vi "TDMS File Initialization (Write).vi"(8 "error in (no error)":errorcluster, 9 "Write Settings":T4={"Asynchronous"=FALSE, "Disable Buffering if Supported"=FALSE, "Reserved Images"=1000, "Fail if Reservation Fails"=FALSE}, 10 "Image In":T5, 11 "File Path":path) -> (0 "error out":errorcluster, 1 "Write Settings Out":T3 {"Image Type" items=["Grayscale (U8)", "Grayscale (I16)", "Grayscale (SGL)", "Complex (CSG)", "RGB (U32)", "HSL (U32)", "RGB (U64)", "Grayscale (U16)"]}, 2 "Optimizations Configured":T1, 3 "TDMS Refnum Out":refnum<k34>)   [LabVIEW 2023]
uses:
  <vilib>/vision/Image Controls.llb/IMAQ Image.ctl
  TDMS Write Settings.ctl
  TDMS Global.vi
  <vilib>/vision/EDVR.llb/IMAQ ImageToEDVR 1D U8.vi
  <vilib>/vision/EDVR.llb/IMAQ ImageToEDVR 1D I16.vi
  <vilib>/vision/EDVR.llb/IMAQ ImageToEDVR 1D U32.vi
  <vilib>/vision/EDVR.llb/IMAQ ImageToEDVR 1D U16.vi
panel:
  # "Overview:  Use this helper VI to initialize the settings for writing TDMS files.\n\nFile Path: Path to Write the file\nImage In: This image is used to initialize write settings for data type and size.\nWrite Settings:\n   Asynchronous: This flag indicates if an asynchronous write should be configured. The asynchronous option produces the most optimized performance, but it's not supported on RT.\n   Disable Buffering if Supported: When the image is a multiple of the sector size, buffering can be disabled, which may improve performance in some cases.  If buffering cannot be disabled, this option is ignored.\n   Reserve Number of Images in File (-1: No Limit): The number of images to reserve  the file for on disk. Reserving the file for the requested number of images can greatly improve performance since disk allocations don't need to happen during the write operation, only once at the beginning. This does require the program to be running with Administrative Privileges and is only allowed on Windows.\n   Fail if Reservation Fails: When this boolean is TRUE, and the number of images to reserve is greater than 0, the VI will fail if the reservation fails. If the boolean is FALSE, the result of the reservation is ignored.  \n\nTDMS Refnum Out: The configured TDMS reference that can be used with TDMS File IO VIs.\nWrite Settings Out: This cluster should be passed to the TDMS Write File helper VI.\n   Image Type:  The image type of the image passed in.\n   Async File Format: Indicates if the write should use the async VIs with the Image Data Value Reference.\nOptimizations Configured: Indicates which optimizations are used.\n   Asynchronous Writes: True when the TDMS session is configured for asynchronous writes.\n   Reserve Disk Space: TRUE when the disk was reserved for the specified number of images.\n   Disable Buffering: TRUE when this option was used."
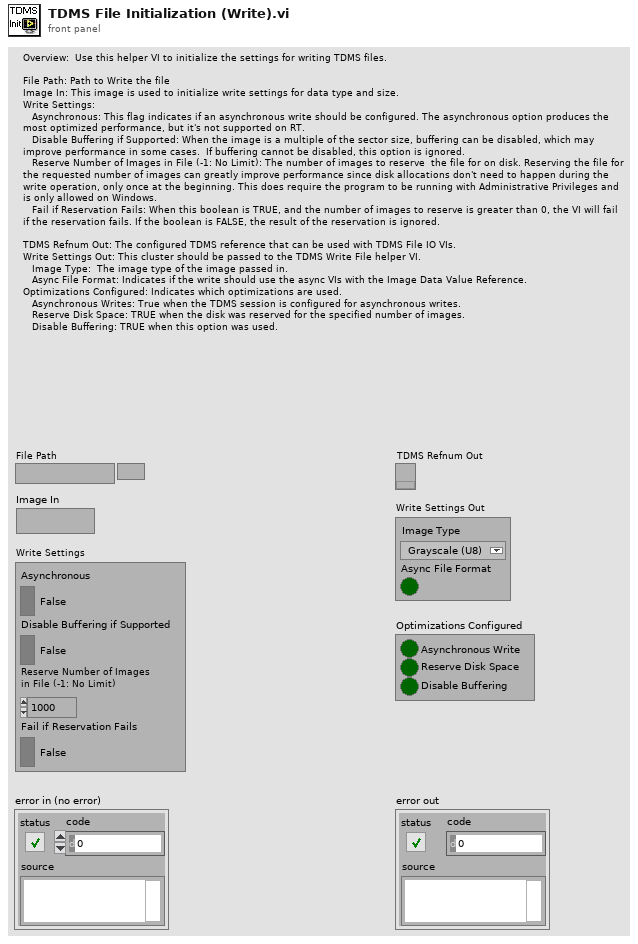
[diagram p1: front panel]
types:
  T1 = cluster{"Asynchronous Write":bool, "Reserve Disk Space":bool, "Disable Buffering":bool}
  T2 = typedef "Image Type" = u32
  T3 = cluster{"Image Type":T2, "Async File Format":bool}
  T4 = typedef "TDMS Write Settings.ctl" = cluster{"Asynchronous":bool, "Disable Buffering if Supported":bool, "Reserved Images":i64, "Fail if Reservation Fails":bool}
  T5 = typedef "IMAQ Image.ctl" = refnum<image>
  T6 = enum16{"open", "open or create", "create or replace", "create", "open (read-only)"}
  T7 = cluster{"Total Width":u32, "Left Border":u32, "Image Data":u32, "Right Border":u32, "Padding":u32}
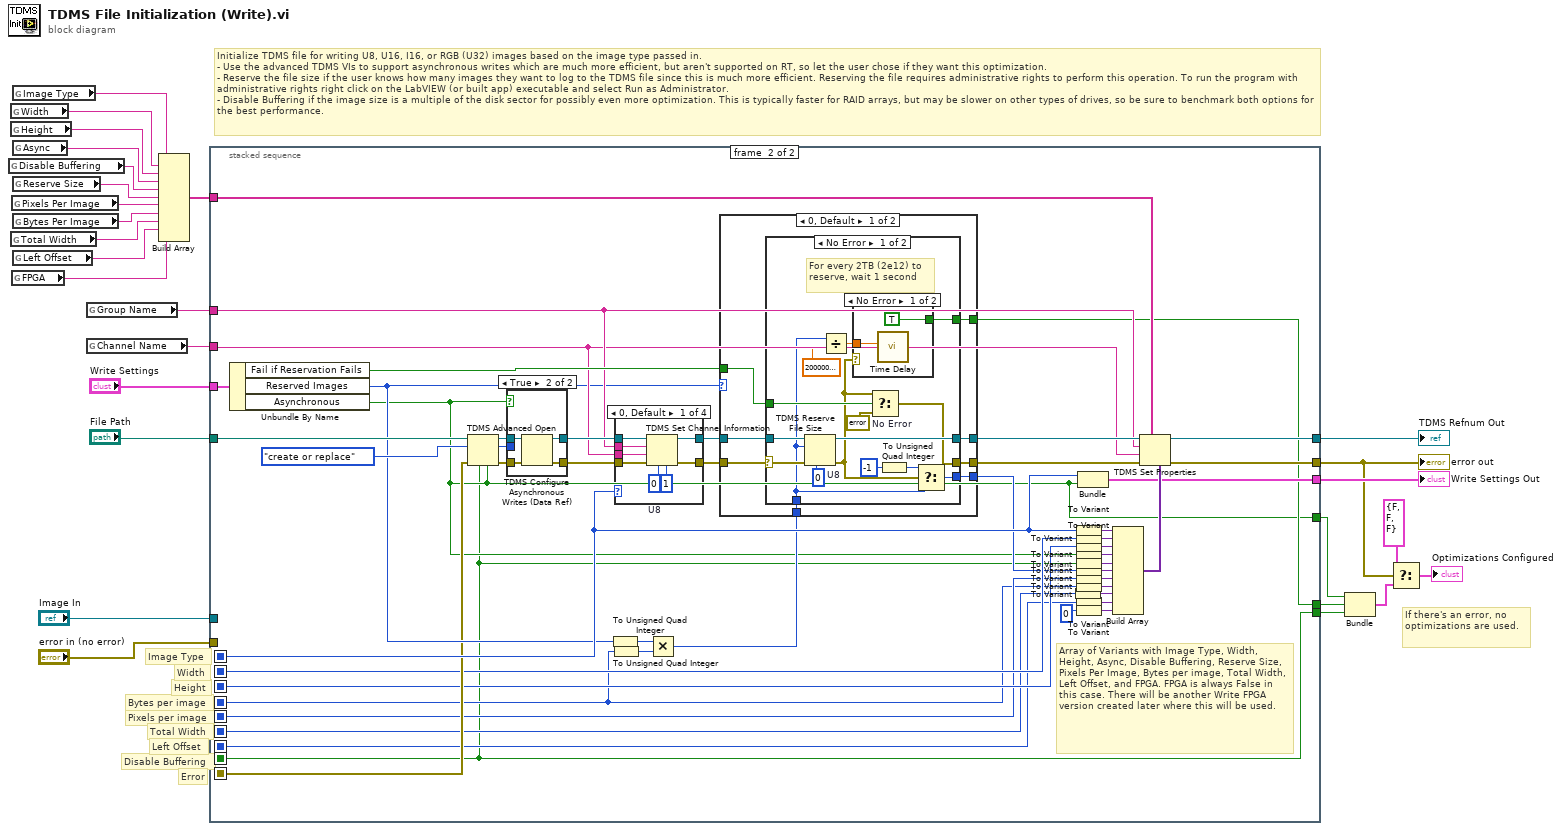
[diagram p0: block diagram]
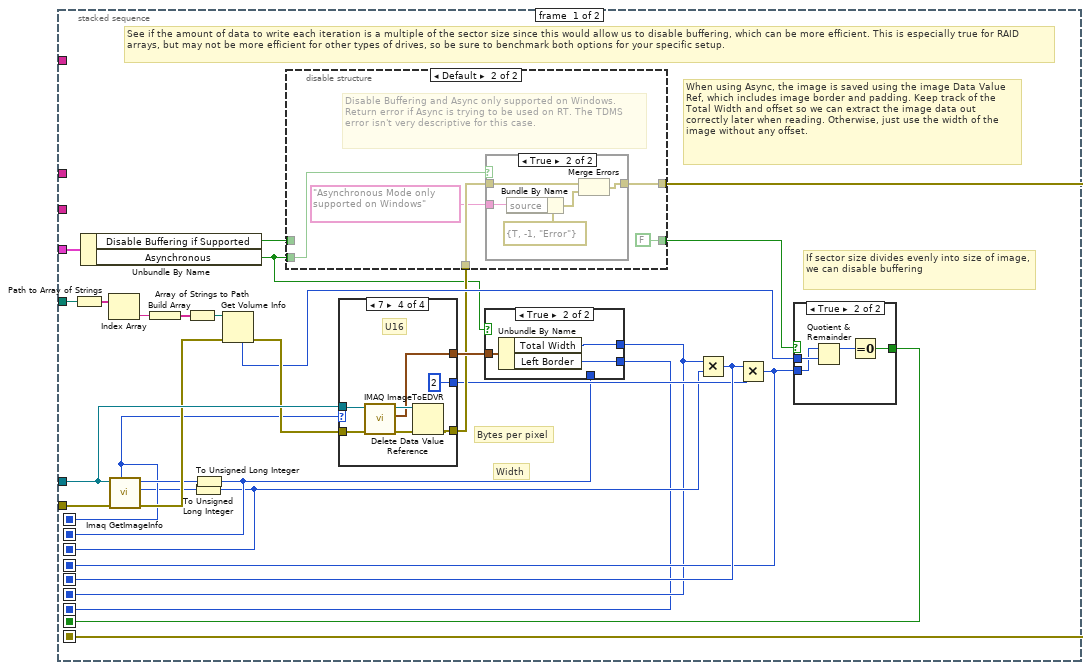
[diagram p2: hidden frame]
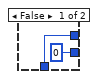
[diagram p3: hidden frame]
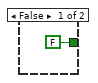
[diagram p4: hidden frame]
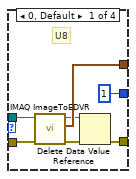
[diagram p7: hidden frame]
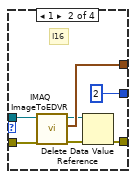
[diagram p8: hidden frame]
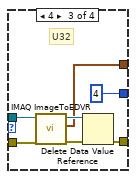
[diagram p9: hidden frame]
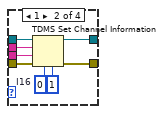
[diagram p14: hidden frame]
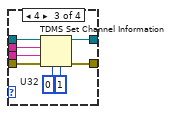
[diagram p15: hidden frame]
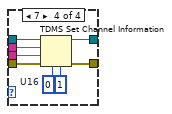
[diagram p16: hidden frame]
diagram:
  # "If there's an error, no optimizations are used."
  # "Total Width"
  # "Error"
  # "Disable Buffering"
  # "Pixels per image"
  # "Bytes per image"
  # "Height"
  # "Width"
  # "Image Type"
  # "Initialize TDMS file for writing U8, U16, I16, or RGB (U32) images based on the image type passed in. \n- Use the advanced TDMS VIs to support asynchronous writes which are much more efficient, but aren't supported on RT, so let the user chose if they want this optimization. \n- Reserve the file size if the user knows how many images they want to log to the TDMS file since this is much more efficient. Reserving the file requires administrative rights to perform this operation. To run the program with administrative rights right click on the LabVIEW (or built app) executable and select Run as Administrator.\n- Disable Buffering if the image size is a multiple of the disk sector for possibly even more optimization. This is typically faster for RAID arrays, but may be slower on other types of drives, so be sure to benchmark both options for the best performance."
  # "Left Offset"
  n1 = global read "TDMS Global.vi" "Disable Buffering"() -> (w10:string)
  n2 = global read "TDMS Global.vi" "Width"() -> (w7:string)
  n3 = global read "TDMS Global.vi" "Height"() -> (w8:string)
  n4 = global read "TDMS Global.vi" "Total Width"() -> (w4:string)
  n5 = global read "TDMS Global.vi" "Pixels Per Image"() -> (w12:string)
  n6 = global read "TDMS Global.vi" "FPGA"() -> (w2:string)
  n7 = global read "TDMS Global.vi" "Image Type"() -> (w6:string)
  n8 = global read "TDMS Global.vi" "Async"() -> (w9:string)
  n9 = global read "TDMS Global.vi" "Reserve Size"() -> (w11:string)
  n10 = global read "TDMS Global.vi" "Bytes Per Image"() -> (w5:string)
  n11 = global read "TDMS Global.vi" "Left Offset"() -> (w3:string)
  n12 = global read "TDMS Global.vi" "Group Name"() -> (w14:string)
  n13 = global read "TDMS Global.vi" "Channel Name"() -> (w13:string)
  n14 = Build Array(w6, w7, w8, w9, w10, w11, w12, w5, w4, w3, w2) -> (w1:string[])
  n15 = stacked-sequence {
    seq-local: [w39 _] -> [_ w107]
    seq-local: [w33 _] -> [_ w118]
    seq-local: [w37 _] -> [_ w126]
    seq-local: [w42 _] -> [_ w130]
    seq-local: [w31 _] -> [_ w124]
    seq-local: [w30 _] -> [_ w123]
    seq-local: [w35 _] -> [_ w119]
    seq-local: [w29 _] -> [_ w117]
    seq-local: [w28 _] -> [_ w116]
    tunnel: w1 -> [_ w147]
    tunnel: "Write Settings" -> [w49 w143]
    tunnel: "error in (no error)" -> [w50 _]
    tunnel: "Image In" -> [w48 _]
    tunnel: [_ w142] -> w27
    tunnel: [_ w141] -> w17
    tunnel: [_ w135] -> w22
    tunnel: w14 -> [_ w134]
    tunnel: w13 -> [_ w133]
    tunnel: "File Path" -> [w51 w131]
    tunnel: [_ w107] -> w21
    tunnel: [_ w108] -> w19
    tunnel: [_ w120] -> w20
    frame #0 {
      # "Bytes per pixel"
      # "Width"
      # "If sector size divides evenly into size of image, we can disable buffering"
      # "When using Async, the image is saved using the image Data Value Ref, which includes image border and padding. Keep track of the Total Width and offset so we can extract the image data out correctly later when reading. Otherwise, just use the width of the image without any offset."
      # "See if the amount of data to write each iteration is a multiple of the sector size since this would allow us to disable buffering, which can be more efficient. This is especially true for RAID arrays, but may not be more efficient for other types of drives, so be sure to benchmark both options for your specific setup."
      n16 = Path to Array of Strings(0:w51) -> (2:w55:string[])  [unwired: 1 out]
      n17 = Unbundle By Name(w49) -> ("Disable Buffering if Supported"=w41:bool, "Asynchronous"=w32:bool)
      n18 = Index Array(array=w55) -> (element=w54:string)  [unwired: 1 in]
      n19 = call "Imaq GetImageInfo"("error in (no error)"=w50, "Image"=w48) -> ("error out"=w47:errorcluster, "Y Resolution"=w36:i32, "X Resolution"=w43:i32, "Image Type"=w42:T2)  [unwired: 2 in, 4 out]
      n20 = Build Array(w54) -> (w53:string[])
      n21 = Array of Strings to Path(0:w53) -> (2:w52:path)  [unwired: 1 in]
      n22 = To Unsigned Long Integer(number=w36) -> (unsigned 32bit integer=w30:u32)
      n23 = To Unsigned Long Integer(number=w43) -> (unsigned 32bit integer=w31:u32)
      n24 = Get Volume Info(8:w47, 11:w52) -> (0:w46:errorcluster, 4:w44:u32)  [unwired: 4 out]
      n25 = case shown="7" w42 {
        tunnel: [u32 1 u32 2 u32 4 u32 2] -> w34
        tunnel: w48 -> [w84 w92 w96 w103]
        tunnel: [w83 w91 w95 w102] -> w45
        tunnel: [w81 w88 w94 w101] -> w38
        tunnel: w46 -> [w80 w86 w93 w100]
        frame 0, Default {
          # "U8"
          n26 = call-poly <vilib>:"IMAQ ImageToEDVR.vi"("error in (no error)"=w80, "Image"=w84) -> ("error out"=w79:errorcluster, "Line Info"=w83:T7, "EDVR 1D U8"=w82:refnum<data-value>)  [unwired: 7 in]
          n27 = Delete Data Value Reference(data value reference=w82, error in=w79) -> (error out=w81:errorcluster)  [unwired: 1 out]
        }
        frame 1 {
          # "I16"
          n28 = call-poly <vilib>:"IMAQ ImageToEDVR.vi"("error in (no error)"=w86, "Image"=w92) -> ("error out"=w89:errorcluster, "Line Info"=w91:T7, "EDVR 1D I16"=w90:refnum<data-value>)  [unwired: 7 in]
          n29 = Delete Data Value Reference(data value reference=w90, error in=w89) -> (error out=w88:errorcluster)  [unwired: 1 out]
        }
        frame 4 {
          # "U32"
          n30 = call-poly <vilib>:"IMAQ ImageToEDVR.vi"("error in (no error)"=w93, "Image"=w96) -> ("error out"=w97:errorcluster, "Line Info"=w95:T7, "EDVR 1D U32"=w98:refnum<data-value>)  [unwired: 7 in]
          n31 = Delete Data Value Reference(data value reference=w98, error in=w97) -> (error out=w94:errorcluster)  [unwired: 1 out]
        }
        frame 7 {
          # "U16"
          n32 = call-poly <vilib>:"IMAQ ImageToEDVR.vi"("error in (no error)"=w100, "Image"=w103) -> ("error out"=w104:errorcluster, "Line Info"=w102:T7, "EDVR 1D U16"=w105:refnum<data-value>)  [unwired: 7 in]
          n33 = Delete Data Value Reference(data value reference=w105, error in=w104) -> (error out=w101:errorcluster)  [unwired: 1 out]
        }
      }
      n34 = disable-structure shown="Default" {
        disable-tunnel: w41 -> [w67 _]
        disable-tunnel: [w67 FALSE ("Disable Buffering if Supported")] -> w40
        disable-tunnel: w32 -> [_ w71]
        disable-tunnel: w38 -> [w66 w70]
        disable-tunnel: [w66 w69] -> w37
        frame condition #0 (active) {
        }
        frame condition #1 {
          # "Disable Buffering and Async only supported on Windows. Return error if Async is trying to be used on RT. The TDMS error isn't very descriptive for this case."
          n35 = case shown="True" w71 {
            tunnel: w70 -> [w73 w77]
            tunnel: [w73 w78] -> w69
            tunnel: "Asynchronous Mode only supported on Windows" ("source") -> [_ w74]
            frame False {
            }
            frame True {
              n36 = Bundle By Name(cluster=errorcluster {"status"=TRUE, "code"=-1, "source"="Error"} ("error in"), "source"=w74) -> (w75:errorcluster)
              n37 = Merge Errors(w77, w75) -> (w78:errorcluster)
            }
          }
        }
      }
      n38 = case shown="True" w32 {
        tunnel: w45 -> [_ w60]
        tunnel: w31 -> [w57 _]
        tunnel: [w57 w59] -> w29
        tunnel: [u32 0 ("Left Border") w58] -> w28
        frame False {
        }
        frame True {
          n39 = Unbundle By Name(w60) -> ("Total Width"=w59:u32, "Left Border"=w58:u32)
        }
      }
      n40 = Multiply(x=w29, y=w30) -> (x*y=w35:u32)
      n41 = Multiply(x=w35, y=w34) -> (x*y=w33:u32)
      n42 = case shown="True" w40 {
        tunnel: w44 -> [_ w65]
        tunnel: [FALSE w63] -> w39
        tunnel: w33 -> [_ w62]
        frame False {
        }
        frame True {
          n43 = Quotient & Remainder(x=w62, y=w65) -> (x-y*floor(x/y)=w64:u32)  [unwired: 1 out]
          n44 = Equal To 0?(x=w64) -> (x = 0?=w63:bool)
        }
      }
    }
    frame #1 {
      # "Array of Variants with Image Type, Width, Height, Async, Disable Buffering, Reserve Size, Pixels Per Image, Bytes per image, Total Width, Left Offset, and FPGA. FPGA is always False in this case. There will be another Write FPGA version created later where this will be used."
      n45 = Unbundle By Name(w143) -> ("Fail if Reservation Fails"=w140:bool, "Reserved Images"=w129:i64, "Asynchronous"=w108:bool)
      n46 = TDMS Advanced Open(4:w108, 6:w107, 8:w126, 10:T6."create or replace" ("operation (0:open)"), 11:w131) -> (0:w151:errorcluster, 2:w132:u32, 3:w150:refnum<k34>)
      n47 = case shown="True" w108 {
        tunnel: [w186 w188] -> w152
        tunnel: w151 -> [w186 w190]
        tunnel: w150 -> [w187 w191]
        tunnel: [w187 w189] -> w148
        tunnel: w132 -> [_ _]
        frame False {
        }
        frame True {
          n48 = TDMS Configure Asynchronous Writes (Data Ref)(8:w190, 11:w191) -> (0:w188:errorcluster, 3:w189:refnum<k34>)  [unwired: 2 in]
        }
      }
      n49 = To Unsigned Quad Integer(1:w129) -> (0:w128:u64)
      n50 = To Unsigned Quad Integer(1:w118) -> (0:w127:u64)
      n51 = case shown="0, Default" w130 {
        tunnel: w148 -> [w199 w207 w215 w223]
        tunnel: [w198 w200 w214 w222] -> w138
        tunnel: w152 -> [w192 w201 w208 w216]
        tunnel: [w196 w205 w212 w220] -> w139
        tunnel: w133 -> [w194 w202 w209 w217]
        tunnel: w134 -> [w193 w203 w210 w218]
        frame 0, Default {
          w195 = u8 0  # U8
          n52 = TDMS Set Channel Information(4:u32 1 ("samples per channel"), 6:w195, 8:w192, 9:w194, 10:w193, 11:w199) -> (0:w198:errorcluster, 3:w196:refnum<k34>)  [unwired: 1 in]
        }
        frame 1 {
          w204 = i16 0  # I16
          n53 = TDMS Set Channel Information(4:u32 1 ("samples per channel"), 6:w204, 8:w201, 9:w202, 10:w203, 11:w207) -> (0:w200:errorcluster, 3:w205:refnum<k34>)  [unwired: 1 in]
        }
        frame 4 {
          w211 = u32 0  # U32
          n54 = TDMS Set Channel Information(4:u32 1 ("samples per channel"), 6:w211, 8:w208, 9:w209, 10:w210, 11:w215) -> (0:w214:errorcluster, 3:w212:refnum<k34>)  [unwired: 1 in]
        }
        frame 7 {
          w219 = u16 0  # U16
          n55 = TDMS Set Channel Information(4:u32 1 ("samples per channel"), 6:w219, 8:w216, 9:w217, 10:w218, 11:w223) -> (0:w222:errorcluster, 3:w220:refnum<k34>)  [unwired: 1 in]
        }
      }
      n56 = Multiply(x=w128, y=w127) -> (x*y=w125:u64)
      n57 = case shown="0, Default" w129 {
        selector: w129 -> [_ w183]
        tunnel: w138 -> [w157 w184]
        tunnel: w139 -> [w162 w185]
        tunnel: [w161 w185] -> w137
        tunnel: [w160 w184] -> w136
        tunnel: w125 -> [w159 _]
        tunnel: w140 -> [w158 _]
        tunnel: [w156 w183] -> w122
        tunnel: [w155 _] -> w120
        frame 0, Default {
          n58 = case shown="No Error" w157 {
            selector: w157 -> [w172 w182]
            tunnel: w162 -> [w177 w181]
            tunnel: [w176 w181] -> w161
            tunnel: [w169 w182] -> w160
            tunnel: w159 -> [w168 w180]
            tunnel: w158 -> [w171 _]
            tunnel: [w167 w180] -> w156
            tunnel: [w163 _] -> w155
            frame No Error {
              w170 = errorcluster {"status"=FALSE, "code"=0, "source"=""}  # No Error
              w175 = u8 0  # U8
              # "For every 2TB (2e12) to reserve, wait 1 second"
              n59 = TDMS Reserve File Size(6:w175, 8:w172, 10:w168, 11:w177) -> (0:w164:errorcluster, 3:w176:refnum<k34>)  [unwired: 1 in]
              n60 = Divide(x=w168, y=2000000000000.0) -> (x/y=w173:dbl)
              n61 = case shown="No Error" w164 {
                tunnel: w173 -> [w179 _]
                tunnel: [TRUE _] -> w163
                frame No Error {
                  n62 = call "Time Delay"("Delay Time (s)"=w179) -> ()  [unwired: 10 in, 1 out]
                }
                frame Error {
                }
              }
              n63 = Select(t=w164, s=w171, f=w170) -> (s? t:f=w169:errorcluster)
              n64 = To Unsigned Quad Integer(1:i64 -1) -> (0:w165:u64)
              n65 = Select(t=w165, s=w164, f=w168) -> (s? t:f=w167:u64)
            }
            frame Error {
            }
          }
        }
        frame ..-1 {
          # "Not reserving disk space"
        }
      }
      n66 = To Variant(anything=w117) -> (Variant=w112:variant)
      n67 = To Variant(anything=w130) -> (Variant=w153:variant)
      n68 = To Variant(anything=w124) -> (Variant=w146:variant)
      n69 = To Variant(anything=w123) -> (Variant=w145:variant)
      n70 = To Variant(anything=w108) -> (Variant=w144:variant)
      n71 = To Variant(anything=w107) -> (Variant=w109:variant)
      n72 = To Variant(anything=w122) -> (Variant=w115:variant)
      n73 = To Variant(anything=w119) -> (Variant=w114:variant)
      n74 = To Variant(anything=w118) -> (Variant=w113:variant)
      n75 = To Variant(anything=w116) -> (Variant=w111:variant)
      n76 = To Variant(anything=0) -> (Variant=w110:variant)
      n77 = Bundle("Image Type"=w130, "Asynchronous"=w108) -> (w135:cluster{"Image Type":T2, "Asynchronous":bool})  [unwired: 1 in]
      n78 = Build Array(w153, w146, w145, w144, w109, w115, w114, w113, w112, w111, w110) -> (w154:variant[])
      n79 = TDMS Set Properties(5:w154, 7:w147, 8:w136, 9:w133, 10:w134, 11:w137) -> (0:w141:errorcluster, 3:w142:refnum<k34>)  [unwired: 2 out]
    }
  }
  "TDMS Refnum Out" <- w27
  "error out" <- w17
  "Write Settings Out" <- w22
  n80 = Bundle("Asynchronous"=w19, w20, w21) -> (w18:cluster{"Asynchronous":bool, bool, bool})  [unwired: 1 in]
  n81 = Select(t=cluster{"Asynchronous":bool, bool, bool} {"Asynchronous"=FALSE, FALSE, FALSE}, s=w17, f=w18) -> (s? t:f=→"Optimizations Configured":cluster{"Asynchronous":bool, bool, bool})
